vi "sub_test-start.vi"(7 "cmd":enum16{"Start", "Finish"}(ring), 8 "error in":errorcluster, 11 "stop?":bool=TRUE) -> (0 "error out":errorcluster)   [LabVIEW 2019]
uses:
  SubVIs/common/_ctrl/system-status.ctl
  _ctrl/rw.ctl
  SubVIs/common/cmd_offtimecheck.ctl
  _ctrl/BP4610_cmd.ctl
  _ctrl/DSP_action.ctl
  SubVIs/cmd_timer.ctl
  SubVIs/count/cmd_count.ctl
  _ctrl/fgv_DL950.ctl
  result.ctl
  shutdown-type.ctl
  _ctrl/init-r-w.ctl
  _ctrl/init-r-stop.ctl
  SubVIs/common/cmd_tablecnt.ctl
  SubVIs/common/Glob_Ref.vi
  Global 1.vi
panel:
  out "logical AND":bool
  out "String":string
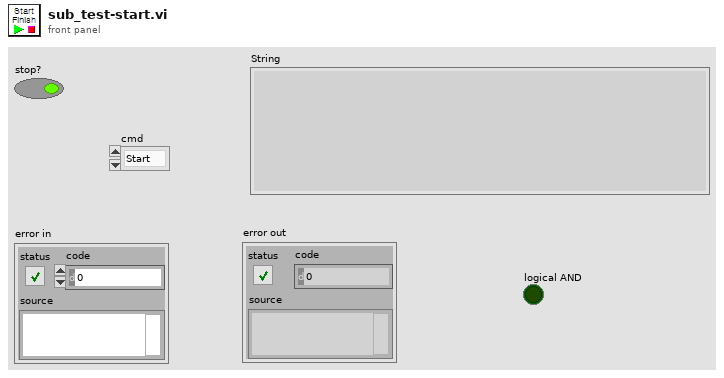
[diagram p1: front panel]
types:
  T1 = typedef "cmd_offtimecheck.ctl" = enum16{"start", "check", "init"}
  T2 = typedef "system-status.ctl" = enum16{"Initial", "Update", "Clear", "Read"}
  T3 = typedef "rw.ctl" = enum16{"read", "write"}
  T4 = typedef "cmd_count.ctl" = enum16{"init", "count", "default"}
  T5 = typedef "cmd_timer.ctl" = enum16{"init", "init_update", "run", "default", "update"}
  T6 = typedef "DSP_action.ctl" = enum16{"False", "cont", "on", "off", "discont", "protection", "protection_seq", "preread", "level_seq", "level_m", "read", "stop", "exit"}
  T7 = typedef "BP4610_cmd.ctl" = enum16{"open", "read", "set", "set_seq", "limit", "limit_seq", "output on", "output off", "close"}
  T8 = enum16{"yellow", "red", "green", "buzz1", "buzz2"}
  T9 = enum8{"Enabled", "Disabled", "Disabled and Grayed Out"}
  T10 = typedef "fgv_DL950.ctl" = enum16{"init", "config", "Set-NCh", "setapply", "trigger", "history_clear", "read", "time-div", "wave-aquis", "start", "query", "abort", "set_items", "reset_items", "read_items", "percent_rise", "trigger_single", "stop", "offset cancel", "close"}
  T11 = typedef "result.ctl" = enum16{"Init", "OK", "NG", "Shutdown", "Testing", "Completion", "Device Error", "Start", "작동", "미작동", "작동 대기", "작동 1"}
  T12 = typedef "shutdown-type.ctl" = enum16{"soft", "all"}
  T13 = typedef "init-r-w.ctl" = enum16{"init", "read", "write"}
  T14 = typedef "init-r-stop.ctl" = enum16{"ini", "read", "stop"}
  T15 = typedef "cmd_tablecnt.ctl" = enum16{"Create", "Inital", "Write", "Default"}
  T16 = typedef "Testing-info.ctl" = cluster{"전체채널수":u8, "현재채널번호":u8, "Irms":dbl, "입력전압":dbl, "입력전류":dbl, "출력전압":dbl, "출력전류":dbl, "온도":dbl, "제어단 단선":bool, "제어단 단락":bool, "제어단 특성변화":bool, "출력단 단선":bool, "출력단 단락":bool, "출력단 특성변화":bool, "출력단 전압":bool, "카운트 일치":bool, "Irms 판정":bool, "온도":bool, "테스트 회수":u32, "TestType":T17, "현재회수":u32, "Ch selection":cluster{"1ch":bool, "2ch":bool, "3ch":bool, "4ch":bool, "5ch":bool, "6ch":bool}, "반복":u32, "Path":path, "파일생성주기":u32, "start time":dbl, "stop time":dbl, "현재반복회수":u32, "NG":cluster{"입출력 카운트":bool, "출력전류RMS":bool}}
  T17 = typedef "sequence_single.ctl" = enum16{"Register", "RC", "B1", "B2", "B3", "Oper_LV", "Oper_HV", "ContR_LV"}
  T18 = typedef "error_rc.ctl" = cluster{"제어단 단선":bool, "제어단 단락":bool, "제어단 특성변화":bool, "출력단 단선":bool, "출력단 단락":bool, "출력단 특성변화":bool, "출력전압":bool, "카운트 일치":bool, "전압 98%":bool, "전압 63%":bool, "전류 37%":bool, "방전전압":bool, "온도":bool}
  T19 = typedef "ref_all.ctl" = cluster{"BP4610 Config":refnum<vi>, "DSP1950 Config":refnum<vi>, "2470-config":refnum<vi>, "cDAQ 9269 AO config":refnum<vi>, "cDAQ 9221 Config":refnum<vi>, "cDAQ-9467 Config":refnum<vi>, "Waveform":refnum<vi>, "DL950 wfm":refnum<vi>, "AI Graph":refnum<vi>, "AO_Wave-config":refnum<vi>, "DL950 items":refnum<vi>, "Volt":refnum<vi>, "Current":refnum<vi>, "AO_Level":refnum<vi>, "RC-Test Judgement ":refnum<vi>, "Log path":refnum<vi>, "시험명":refnum<vi>, "file renew[Hr]":refnum<vi>, "Breakdown-Spec":refnum<vi>, "paste":refnum<vi>, "copy":refnum<vi>, "DL950_config":refnum<vi>, "종료시간":refnum<vi>, "경과시간":refnum<vi>, "Apply":refnum<vi>, "DSP Config LV ":refnum<vi>, "Testconfig":refnum<vi>}
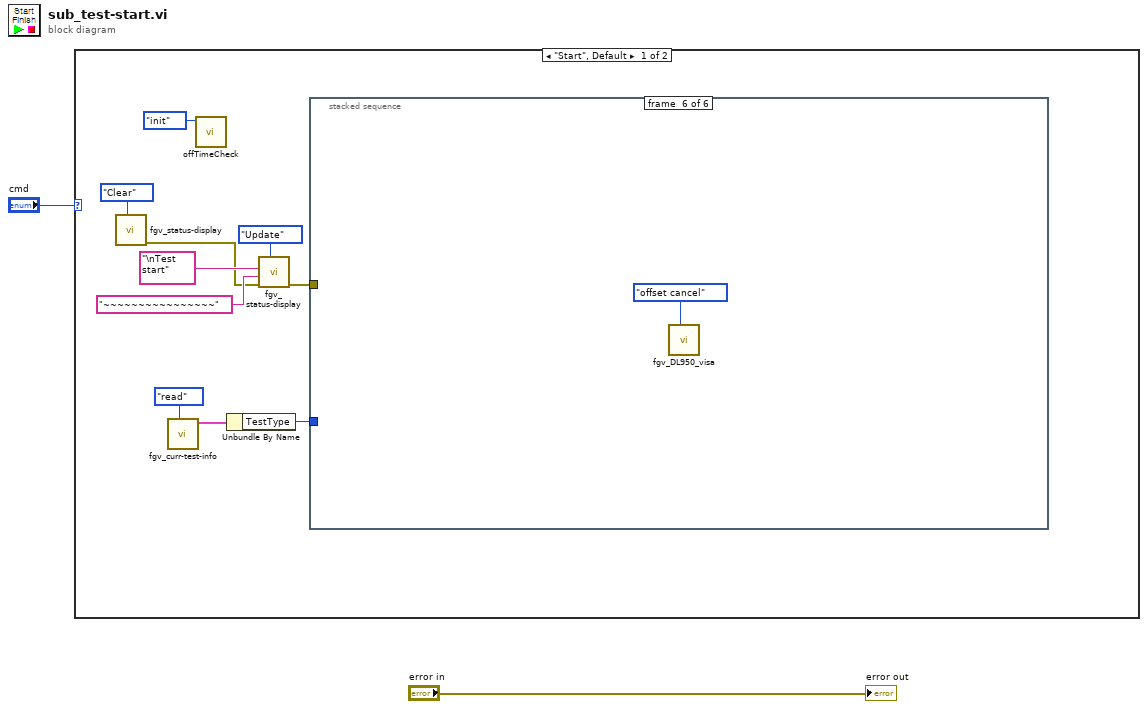
[diagram p0: block diagram]
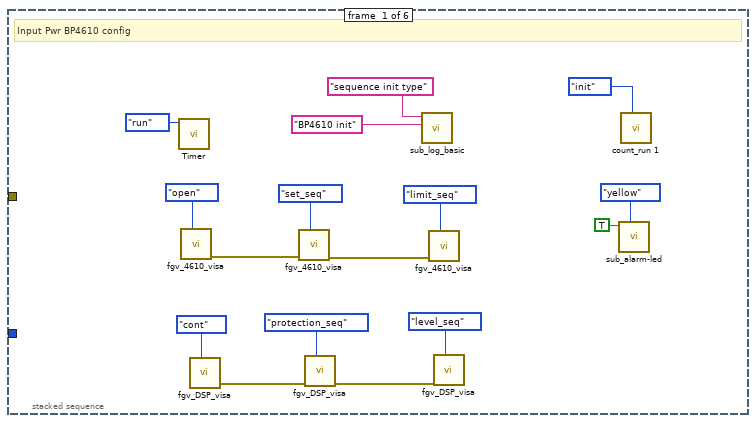
[diagram p2: hidden frame]
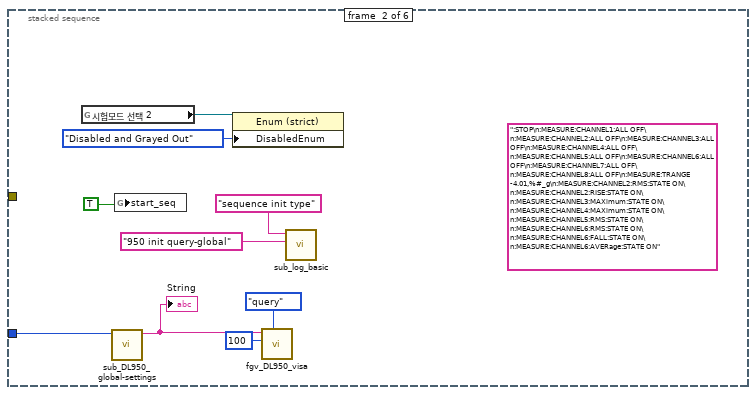
[diagram p3: hidden frame]
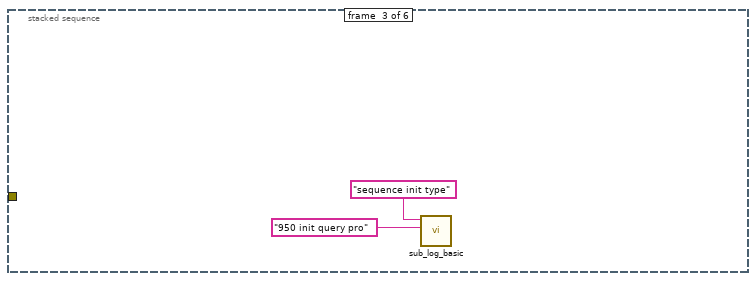
[diagram p4: hidden frame]
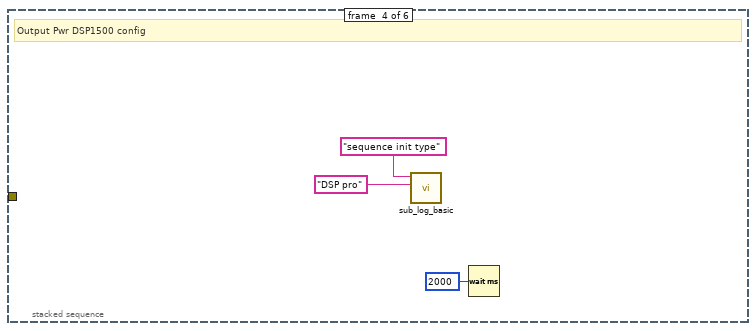
[diagram p5: hidden frame]
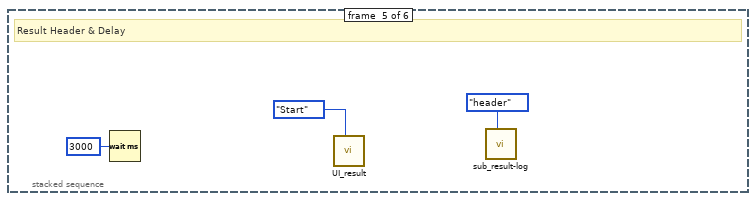
[diagram p6: hidden frame]
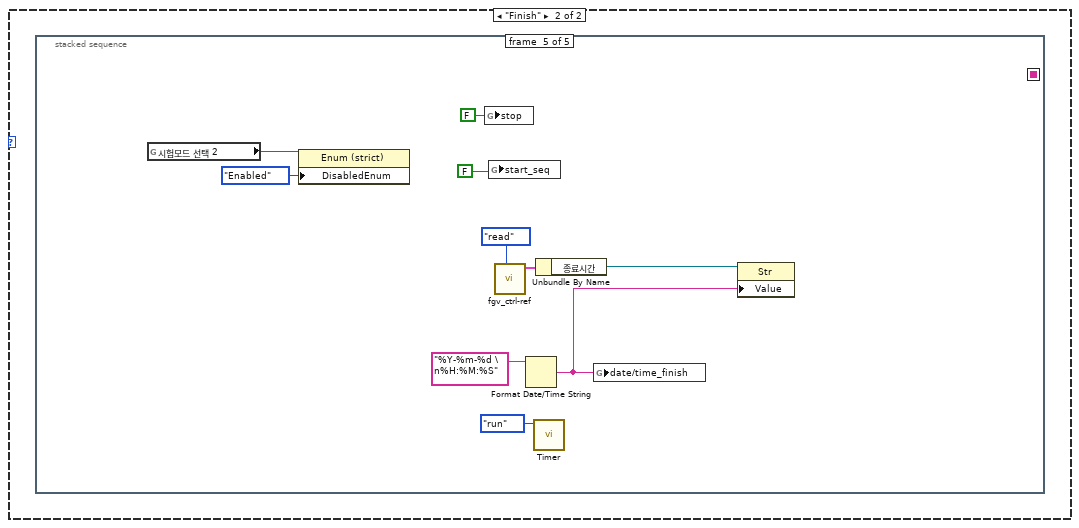
[diagram p7: hidden frame]
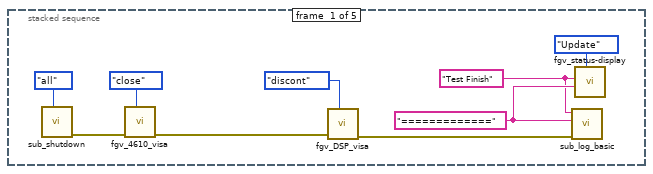
[diagram p8: hidden frame]
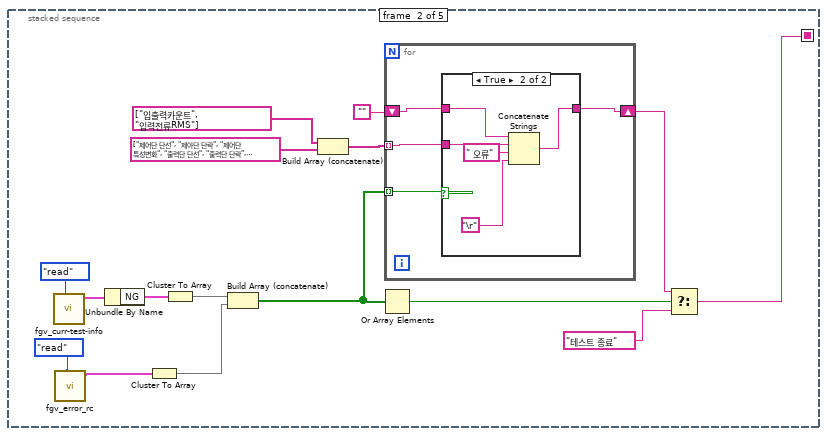
[diagram p9: hidden frame]
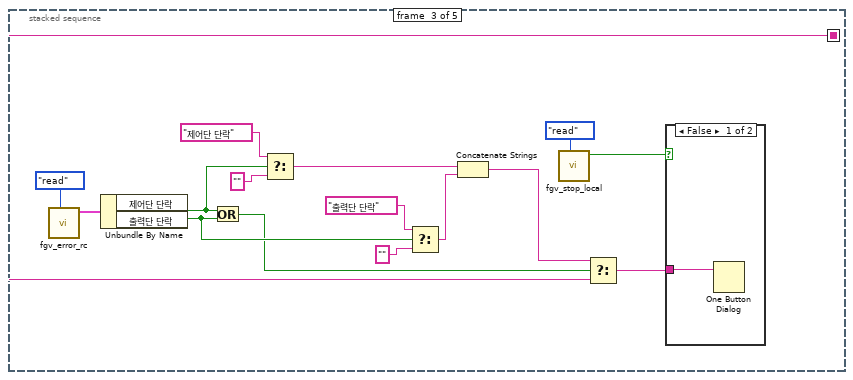
[diagram p11: hidden frame]
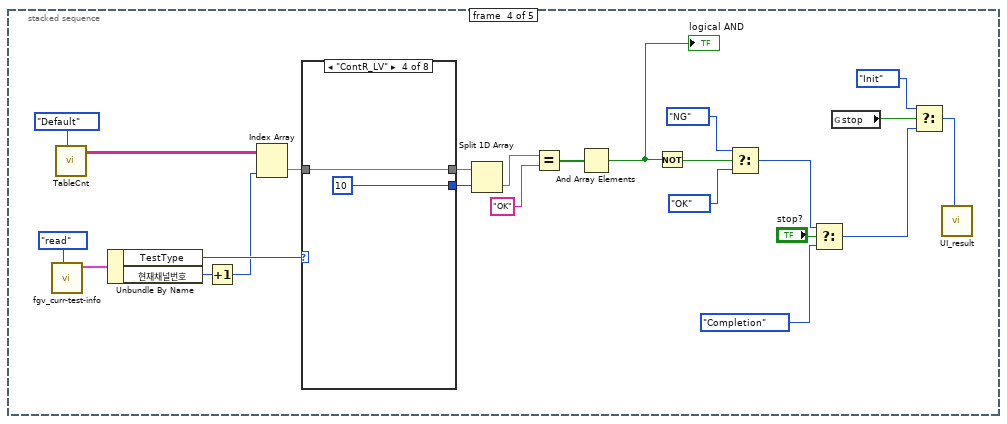
[diagram p13: hidden frame]
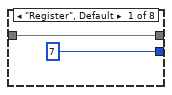
[diagram p14: hidden frame]
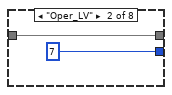
[diagram p15: hidden frame]
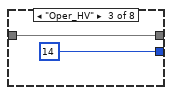
[diagram p16: hidden frame]
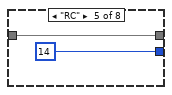
[diagram p17: hidden frame]
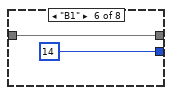
[diagram p18: hidden frame]
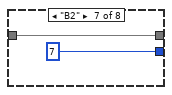
[diagram p19: hidden frame]
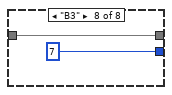
[diagram p20: hidden frame]
diagram:
  n1 = case shown="\"Start\", Default" "cmd" {
    frame "Start", Default {
      n2 = call "fgv_status-display.vi"("Mode"=system-status."Clear") -> ("error out"=w4:errorcluster)  [unwired: 10 in]
      n3 = call "fgv_curr-test-info.vi"("cmd"=rw."read") -> ("현재테스트 정보 2"=w9:T16)  [unwired: 10 in]
      n4 = call "offTimeCheck.vi"("cmd"=cmd_offtimecheck."init") -> ()  [unwired: 10 in, 1 out]
      n5 = Unbundle By Name(w9) -> ("TestType"=w6:T17)
      n6 = call "fgv_status-display.vi"("Mode"=system-status."Update", "error in"=w4, "detail"="~~~~~~~~~~~~~~~~", "title"="\nTest start" ("Title")) -> ("error out"=w7:errorcluster)  [unwired: 7 in]
      n7 = stacked-sequence {
        tunnel: w6 -> [_ w37 _ _ _ _]
        tunnel: w7 -> [_ _ _ _ _ _]
        frame #0 {
          # "Input Pwr BP4610 config"
          n8 = call "Timer.vi"("cmd"=cmd_timer."run") -> ()  [unwired: 8 in, 3 out]
          n9 = call "fgv_4610_visa.vi"("cmd"=BP4610_cmd."open") -> ("error out"=w23:errorcluster)  [unwired: 10 in]
          n10 = call "fgv_DSP_visa.vi"("action"=DSP_action."cont") -> ("error out"=w19:errorcluster)  [unwired: 10 in]
          n11 = call "fgv_4610_visa.vi"("cmd"=BP4610_cmd."set_seq", "error in"=w23) -> ("error out"=w24:errorcluster)  [unwired: 9 in]
          n12 = call "fgv_DSP_visa.vi"("action"=DSP_action."protection_seq", "error in"=w19) -> ("error out"=w15:errorcluster)  [unwired: 9 in]
          n13 = call "sub_log_basic.vi"("desc"="BP4610 init", "Title"="sequence init type") -> ()  [unwired: 9 in, 1 out]
          n14 = call "fgv_4610_visa.vi"("cmd"=BP4610_cmd."limit_seq", "error in"=w24) -> ()  [unwired: 9 in, 1 out]
          n15 = call "fgv_DSP_visa.vi"("action"=DSP_action."level_seq", "error in"=w15) -> ()  [unwired: 9 in, 1 out]
          n16 = call "sub_alarm-led.vi"("alarm"=T8."yellow", "onoff"=TRUE) -> ()  [unwired: 9 in, 1 out]
          n17 = call "count_run 1.vi"("cmd"=cmd_count."init") -> ()  [unwired: 9 in, 2 out]
        }
        frame #1 {
          (unwired) ":STOP\n:MEASURE:CHANNEL1:ALL OFF\n:MEASURE:CHANNEL2:ALL OFF\n:MEASURE:CHANNEL3:ALL OFF\n:MEASURE:CHANNEL4:ALL OFF\n:MEASURE:CHANNEL5:ALL OFF\n:MEASURE:CHANNEL6:ALL OFF\n:MEASURE:CHANNEL7:ALL OFF\n:MEASURE:CHANNEL8:ALL OFF\n:MEASURE:TRANGE -4.01,%#_g\n:MEASURE:CHANNEL2:RMS:STATE ON\n:MEASURE:CHANNEL2:RISE:STATE ON\n:MEASURE:CHANNEL3:MAXimum:STATE ON\n:MEASURE:CHANNEL4:MAXimum:STATE ON\n:MEASURE:CHANNEL5:RMS:STATE ON\n:MEASURE:CHANNEL6:RMS:STATE ON\n:MEASURE:CHANNEL6:FALL:STATE ON\n:MEASURE:CHANNEL6:AVERage:STATE ON" ("String")
          n18 = global read "Global 1.vi" "시험모드 선택 2"() -> (w30:refnum<vi>)
          n19 = call "sub_DL950_global-settings.vi"("TestType"=w37) -> ("String"=w31:string)  [unwired: 10 in]
          "String" <- w31
          n20 = global write "Glob_Ref.vi" "start_seq"(TRUE ("stop")) -> ()
          n21 = property class="Enum (strict)"(reference=w30, "DisabledEnum"=T9."Disabled and Grayed Out" ("Disabled")) -> ()  [unwired: 1 in, 2 out]
          n22 = call "fgv_DL950_visa.vi"("cmd"=fgv_DL950."query", "ms"=u32 100, "Initiate"=w31) -> ()  [unwired: 6 in, 3 out]
          n23 = call "sub_log_basic.vi"("desc"="950 init query-global", "Title"="sequence init type") -> ()  [unwired: 9 in, 1 out]
        }
        frame #2 {
          n24 = call "sub_log_basic.vi"("desc"="950 init query pro", "Title"="sequence init type") -> ()  [unwired: 9 in, 1 out]
        }
        frame #3 {
          # "Output Pwr DSP1500 config"
          n25 = call "sub_log_basic.vi"("desc"="DSP pro", "Title"="sequence init type") -> ()  [unwired: 9 in, 1 out]
          n26 = Wait (ms)(milliseconds to wait=u32 2000) -> ()  [unwired: 1 out]
        }
        frame #4 {
          # "Result Header & Delay"
          n27 = Wait (ms)(milliseconds to wait=u32 3000) -> ()  [unwired: 1 out]
          n28 = call "UI_result.vi"("result"=result."Start") -> ()  [unwired: 10 in, 1 out]
          n29 = call "sub_result-log.vi"("data"=enum16{"header", "result"}."header") -> ()  [unwired: 11 in]
        }
        frame #5 {
          n30 = call "fgv_DL950_visa.vi"("cmd"=fgv_DL950."offset cancel") -> ()  [unwired: 8 in, 3 out]
        }
      }
    }
    frame "Finish" {
      n31 = stacked-sequence {
        seq-local: [_ w56 _ _ _] -> [_ _ w82 _ _]
        frame #0 {
          w54 = "=============" ("desc")
          w53 = "Test Finish" ("Title")
          n32 = call "sub_shutdown.vi"("type"=shutdown-type."all") -> ("error out"=w51:errorcluster)  [unwired: 10 in]
          n33 = call "fgv_4610_visa.vi"("cmd"=BP4610_cmd."close", "error in"=w51) -> ("error out"=w52:errorcluster)  [unwired: 9 in]
          n34 = call "fgv_DSP_visa.vi"("action"=DSP_action."discont", "error in"=w52) -> ("error out"=w47:errorcluster)  [unwired: 9 in]
          n35 = call "sub_log_basic.vi"("error in"=w47, "desc"=w54, "Title"=w53) -> ()  [unwired: 8 in, 1 out]
          n36 = call "fgv_status-display.vi"("Mode"=system-status."Update", "detail"=w54, "title"=w53) -> ()  [unwired: 8 in, 1 out]
        }
        frame #1 {
          n37 = call "fgv_curr-test-info.vi"("cmd"=rw."read") -> ("현재테스트 정보 2"=w67:T16)  [unwired: 10 in]
          n38 = call "fgv_error_rc.vi"("cmd"=init-r-w."read") -> ("Error 2"=w64:T18)  [unwired: 10 in]
          n39 = Unbundle By Name(w67) -> ("NG"=w68:cluster{"입출력 카운트":bool, "출력전류RMS":bool})
          n40 = Cluster To Array(cluster=w64) -> (array=w57:bool[])
          n41 = Cluster To Array(cluster=w68) -> (array=w69:bool[])
          n42 = Build Array (concatenate)(w69, w57) -> (w70:bool[])
          n43 = Build Array (concatenate)(string[] ["입출력카운트", "입력전류RMS"], string[] ["제어단 단선", "제아단 단락", "제어단 특성변화", "출력단 단선", "출력단 단락", "출력단 특성변화", "출력전압", "카운트 일치", "전압 98%", "전압 63%", "전류 37%", "방전전압", "온도"]) -> (w71:string[])
          n44 = Or Array Elements(Boolean array=w70) -> (logical OR=w65:bool)
          n45 = for {
            tunnel: w71 -> [w72] mode=indexing
            tunnel: w70 -> [w73] mode=indexing
            shift-right: [w75] -> w66
            shift-left: "" -> [w74]
            n46 = case shown="True" w73 {
              tunnel: [w76 w80] -> w75
              tunnel: w74 -> [w76 w81]
              tunnel: w72 -> [_ w79]
              frame False {
              }
              frame True {
                n47 = Concatenate Strings(w81, w79, " 오류" ("string"), "\r") -> (w80:string)
              }
            }
          }
          n48 = Select(t=w66, s=w65, f="테스트 종료" ("message")) -> (s? t:f=w56:string)
        }
        frame #2 {
          n49 = call "fgv_error_rc.vi"("cmd"=init-r-w."read") -> ("Error 2"=w89:T18)  [unwired: 10 in]
          n50 = Unbundle By Name(w89) -> ("제어단 단락"=w91:bool, "출력단 단락"=w93:bool)
          n51 = Or(x=w91, y=w93) -> (x .or. y?=w90:bool)
          n52 = Select(t="제어단 단락" ("Title"), s=w91, f="" ("Title")) -> (s? t:f=w92:string)
          n53 = Select(t="출력단 단락" ("Title"), s=w93, f="" ("Title")) -> (s? t:f=w94:string)
          n54 = Concatenate Strings(w92, w94) -> (w95:string)
          n55 = call "fgv_stop_local.vi"("cmd"=init-r-stop."read") -> ("stop"=w97:bool)  [unwired: 9 in, 1 out]
          n56 = Select(t=w95, s=w90, f=w82) -> (s? t:f=w96:string)
          n57 = case shown="False" w97 {
            tunnel: w96 -> [w98 _]
            frame False {
              n58 = One Button Dialog(message=w98) -> ()  [unwired: 1 in, 1 out]
            }
            frame True {
            }
          }
        }
        frame #3 {
          n59 = call "fgv_curr-test-info.vi"("cmd"=rw."read") -> ("현재테스트 정보 2"=w112:T16)  [unwired: 10 in]
          n60 = call "TableCnt.vi"("cnt"=cmd_tablecnt."Default") -> ("Item Names"=w110:string[][])  [unwired: 9 in, 1 out]
          n61 = Unbundle By Name(w112) -> ("TestType"=w109:T17, "현재채널번호"=w108:u8)
          n62 = Increment(x=w108) -> (x+1=w107:u8)
          n63 = Index Array(array=w110, index (col)=w107) -> (element=w105:string[])  [unwired: 1 in]
          n64 = case shown="\"ContR_LV\"" w109 {
            tunnel: [w124 w126 w128 w130 w132 w133 w136 w138] -> w106
            tunnel: w105 -> [w124 w126 w128 w130 w132 w133 w136 w138]
            tunnel: [7 ("y") 7 ("y") 14 ("y") 10 ("y") 14 ("y") 14 ("y") 7 ("y") 7 ("y")] -> w104
            frame "Register", Default {
            }
            frame "Oper_LV" {
            }
            frame "Oper_HV" {
            }
            frame "ContR_LV" {
            }
            frame "RC" {
            }
            frame "B1" {
            }
            frame "B2" {
            }
            frame "B3" {
            }
          }
          n65 = Split 1D Array(array=w106, index=w104) -> (second subarray=w119:string[])  [unwired: 1 out]
          n66 = Equal?(x=w119, y="OK" ("message")) -> (x = y?=w120:bool[])
          n67 = And Array Elements(Boolean array=w120) -> (logical AND=w122:bool)
          "logical AND" <- w122
          n68 = Not(x=w122) -> (.not. x?=w121:bool)
          n69 = Select(t=result."NG" ("result"), s=w121, f=result."OK" ("result")) -> (s? t:f=w102:T11)
          n70 = Select(t=w102, s="stop?", f=result."Completion" ("result")) -> (s? t:f=w100:T11)
          n71 = global read "Glob_Ref.vi" "stop"() -> (w115:bool)
          n72 = Select(t=result."Init" ("result"), s=w115, f=w100) -> (s? t:f=w99:T11)
          n73 = call "UI_result.vi"("result"=w99) -> ()  [unwired: 10 in, 1 out]
        }
        frame #4 {
          n74 = global read "Global 1.vi" "시험모드 선택 2"() -> (w140:refnum<vi>)
          n75 = property class="Enum (strict)"(reference=w140, "DisabledEnum"=T9."Enabled" ("Disabled")) -> ()  [unwired: 1 in, 2 out]
          n76 = global write "Glob_Ref.vi" "stop"(FALSE ("stop")) -> ()
          n77 = global write "Glob_Ref.vi" "start_seq"(FALSE ("stop")) -> ()
          n78 = call "fgv_ctrl-ref.vi"("cmd"=rw."read") -> ("output cluster 2"=w145:T19)  [unwired: 9 in, 1 out]
          n79 = Format Date/Time String(time format string (%c)="%Y-%m-%d \n%H:%M:%S" ("시간 포맷 문자열 (%c)")) -> (date/time string=w142:string)  [unwired: 2 in]
          n80 = call "Timer.vi"("cmd"=cmd_timer."run") -> ()  [unwired: 8 in, 3 out]
          n81 = Unbundle By Name(w145) -> ("종료시간"=w144:refnum<vi>)
          n82 = global write "Glob_Ref.vi" "date/time_finish"(w142) -> ()
          n83 = property class="Str"(reference=w144, "Value"=w142) -> ()  [unwired: 1 in, 2 out]
        }
      }
    }
  }
  "error out" <- "error in"
